vi "FlatToRichnixnet_grpc_DisconnectTerminalsRequest.vi"(5 "OutputClusterType":T1, 11 "InputCluster":T3) -> (3 "OutputCluster":T1)   [LabVIEW 2025, in "xnet-grpc_client.lvlib"]
uses:
  nixnet_grpc_DisconnectTerminalsRequest_Flat.ctl
  nidevice_grpc_Session_Flat.ctl
  nixnet_grpc_TerminalName.ctl
  nixnet_grpc_DisconnectTerminalsRequest.ctl
  nixnet_grpc_DisconnectTerminalsRequest_source_enum/nixnet_grpc_DisconnectTerminalsRequest_source_enum.lvclass
  nixnet_grpc_DisconnectTerminalsRequest_destination_enum/nixnet_grpc_DisconnectTerminalsRequest_destination_enum.lvclass
  nidevice_grpc_Session.ctl
  xnet-grpc_client.lvlib
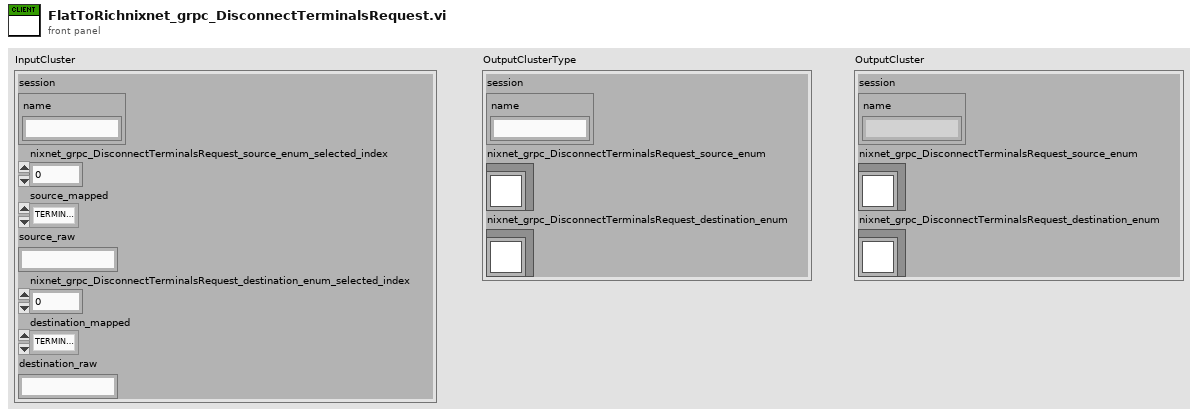
[diagram p1: front panel]
types:
  T1 = typedef "xnet-grpc_client.lvlib/nixnet_grpc_DisconnectTerminalsRequest.ctl" = cluster{"session":T2, "nixnet_grpc_DisconnectTerminalsRequest_source_enum":refnum<class "nixnet_grpc_DisconnectTerminalsRequest_source_enum.lvclass">, "nixnet_grpc_DisconnectTerminalsRequest_destination_enum":refnum<class "nixnet_grpc_DisconnectTerminalsRequest_destination_enum.lvclass">}
  T2 = typedef "xnet-grpc_client.lvlib/nidevice_grpc_Session.ctl" = cluster{"name":string}
  T3 = typedef "xnet-grpc_client.lvlib/nixnet_grpc_DisconnectTerminalsRequest_Flat.ctl" = cluster{"session":T4, "nixnet_grpc_DisconnectTerminalsRequest_source_enum_selected_index":i32, "source_mapped":T5, "source_raw":string, "nixnet_grpc_DisconnectTerminalsRequest_destination_enum_selected_index":i32, "destination_mapped":T5, "destination_raw":string}
  T4 = typedef "xnet-grpc_client.lvlib/nidevice_grpc_Session_Flat.ctl" = cluster{"name":string}
  T5 = typedef "xnet-grpc_client.lvlib/nixnet_grpc_TerminalName.ctl" = enum32{"TERMINAL_NAME_UNSPECIFIED", "TERMINAL_NAME_PXI_TRIG_0", "TERMINAL_NAME_PXI_TRIG_1", "TERMINAL_NAME_PXI_TRIG_2", "TERMINAL_NAME_PXI_TRIG_3", "TERMINAL_NAME_PXI_TRIG_4", "TERMINAL_NAME_PXI_TRIG_5", "TERMINAL_NAME_PXI_TRIG_6", "TERMINAL_NAME_PXI_TRIG_7", "TERMINAL_NAME_FRONT_PANEL_0", "TERMINAL_NAME_FRONT_PANEL_1", "TERMINAL_NAME_PXI_STAR", "TERMINAL_NAME_PXI_CLK_10", "TERMINAL_NAME_10_MHZ_TIMEBASE", "TERMINAL_NAME_1_MHZ_TIMEBASE", "TERMINAL_NAME_MASTER_TIMEBASE", "TERMINAL_NAME_COMM_TRIGGER", "TERMINAL_NAME_START_TRIGGER", "TERMINAL_NAME_FLEX_RAY_START_CYCLE", "TERMINAL_NAME_FLEX_RAY_MACROTICK", "TERMINAL_NAME_LOG_TRIGGER", "TERMINAL_NAME_TIME_TRIGGER", "TERMINAL_NAME_NETWORK_TIME_PPS", "TERMINAL_NAME_NETWORK_TIME_1_MHZ"}
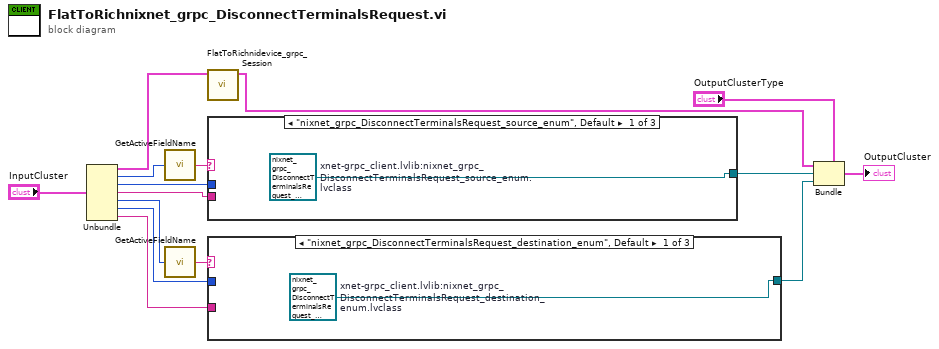
[diagram p0: block diagram]
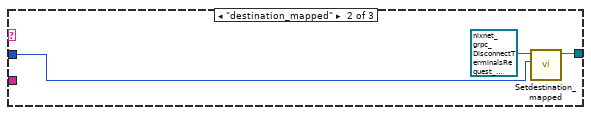
[diagram p2: hidden frame]
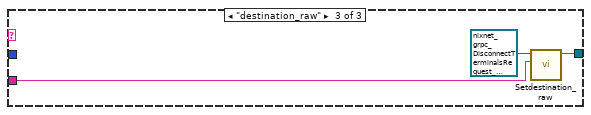
[diagram p3: hidden frame]
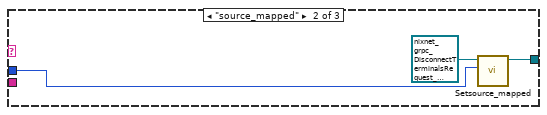
[diagram p4: hidden frame]
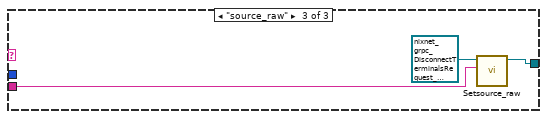
[diagram p5: hidden frame]
diagram:
  n1 = Unbundle "Unbundle"("InputCluster") -> ("session"=w12:T4, "nixnet_grpc_DisconnectTerminalsRequest_source_enum_selected_index"=w10:i32, "source_mapped"=w7:T5, "source_raw"=w6:string, "nixnet_grpc_DisconnectTerminalsRequest_destination_enum_selected_index"=w5:i32, "destination_mapped"=w2:T5, "destination_raw"=w1:string)
  n2 = call "GetActiveFieldName.vi"("protobuf index"=w10) -> ("oneof field name"=w9:string)
  n3 = call "GetActiveFieldName.vi"("protobuf index"=w5) -> ("oneof field name"=w4:string)
  n4 = call "FlatToRichnidevice_grpc_Session.vi"("InputCluster"=w12) -> ("OutputCluster"=w11:T2)  [unwired: 10 in]
  n5 = case "nixnet_grpc_DisconnectTerminalsRequest_source_enum" shown="\"nixnet_grpc_DisconnectTerminalsRequest_source_enum\", Default" w9 {
    tunnel: [w16 w18 w21] -> w8
    tunnel: w7 -> [_ w19 _]
    tunnel: w6 -> [_ _ w22]
    frame "nixnet_grpc_DisconnectTerminalsRequest_source_enum", Default {
      w16 = refnum<class "nixnet_grpc_DisconnectTerminalsRequest_source_enum.lvclass"> refnum  # xnet-grpc_client.lvlib:nixnet_grpc_DisconnectTerminalsRequest_source_enum.lvclass
    }
    frame "source_mapped" {
      n6 = call "Setsource_mapped.vi"("Set_Val"=w19, "OneOfTemplate in"=refnum<class "nixnet_grpc_DisconnectTerminalsRequest_source_enum.lvclass"> refnum) -> ("OneOfTemplate out"=w18:refnum<class "nixnet_grpc_DisconnectTerminalsRequest_source_enum.lvclass">)  [unwired: 8 in, 1 out]
    }
    frame "source_raw" {
      n7 = call "Setsource_raw.vi"("Set_Val"=w22, "OneOfTemplate in"=refnum<class "nixnet_grpc_DisconnectTerminalsRequest_source_enum.lvclass"> refnum) -> ("OneOfTemplate out"=w21:refnum<class "nixnet_grpc_DisconnectTerminalsRequest_source_enum.lvclass">)  [unwired: 8 in, 1 out]
    }
  }
  n8 = case "nixnet_grpc_DisconnectTerminalsRequest_destination_enum" shown="\"nixnet_grpc_DisconnectTerminalsRequest_destination_enum\", Default" w4 {
    tunnel: [w23 w25 w28] -> w3
    tunnel: w2 -> [_ w26 _]
    tunnel: w1 -> [_ _ w29]
    frame "nixnet_grpc_DisconnectTerminalsRequest_destination_enum", Default {
      w23 = refnum<class "nixnet_grpc_DisconnectTerminalsRequest_destination_enum.lvclass"> refnum  # xnet-grpc_client.lvlib:nixnet_grpc_DisconnectTerminalsRequest_destination_enum.lvclass
    }
    frame "destination_mapped" {
      n9 = call "Setdestination_mapped.vi"("Set_Val"=w26, "OneOfTemplate in"=refnum<class "nixnet_grpc_DisconnectTerminalsRequest_destination_enum.lvclass"> refnum) -> ("OneOfTemplate out"=w25:refnum<class "nixnet_grpc_DisconnectTerminalsRequest_destination_enum.lvclass">)  [unwired: 8 in, 1 out]
    }
    frame "destination_raw" {
      n10 = call "Setdestination_raw.vi"("Set_Val"=w29, "OneOfTemplate in"=refnum<class "nixnet_grpc_DisconnectTerminalsRequest_destination_enum.lvclass"> refnum) -> ("OneOfTemplate out"=w28:refnum<class "nixnet_grpc_DisconnectTerminalsRequest_destination_enum.lvclass">)  [unwired: 8 in, 1 out]
    }
  }
  n11 = Bundle "Bundle"(cluster="OutputClusterType", "session"=w11, "nixnet_grpc_DisconnectTerminalsRequest_source_enum"=w8, "nixnet_grpc_DisconnectTerminalsRequest_destination_enum"=w3) -> (→"OutputCluster":T1)
